vi "Navigation plus.vi"(11 "Array":dbl[](array[numeric])) -> (2 "length":i32, 3 "String":string)   [LabVIEW 2021]
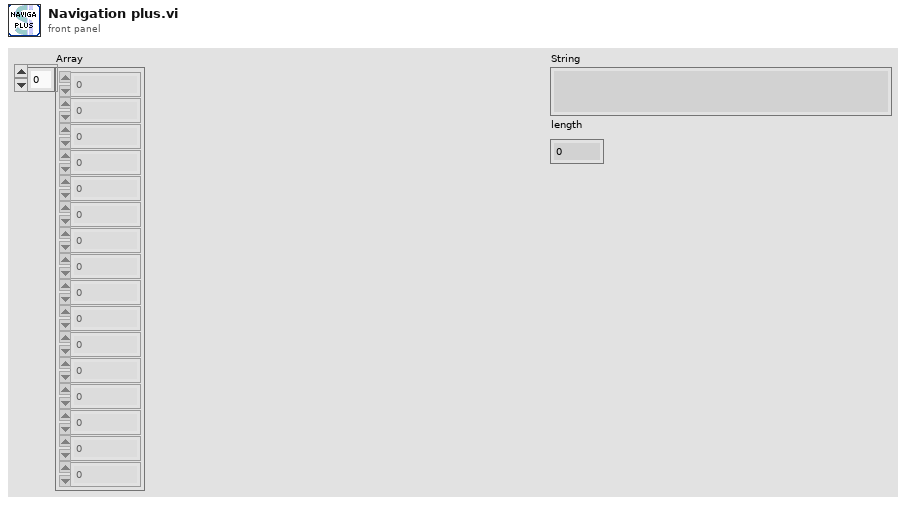
[diagram p1: front panel]
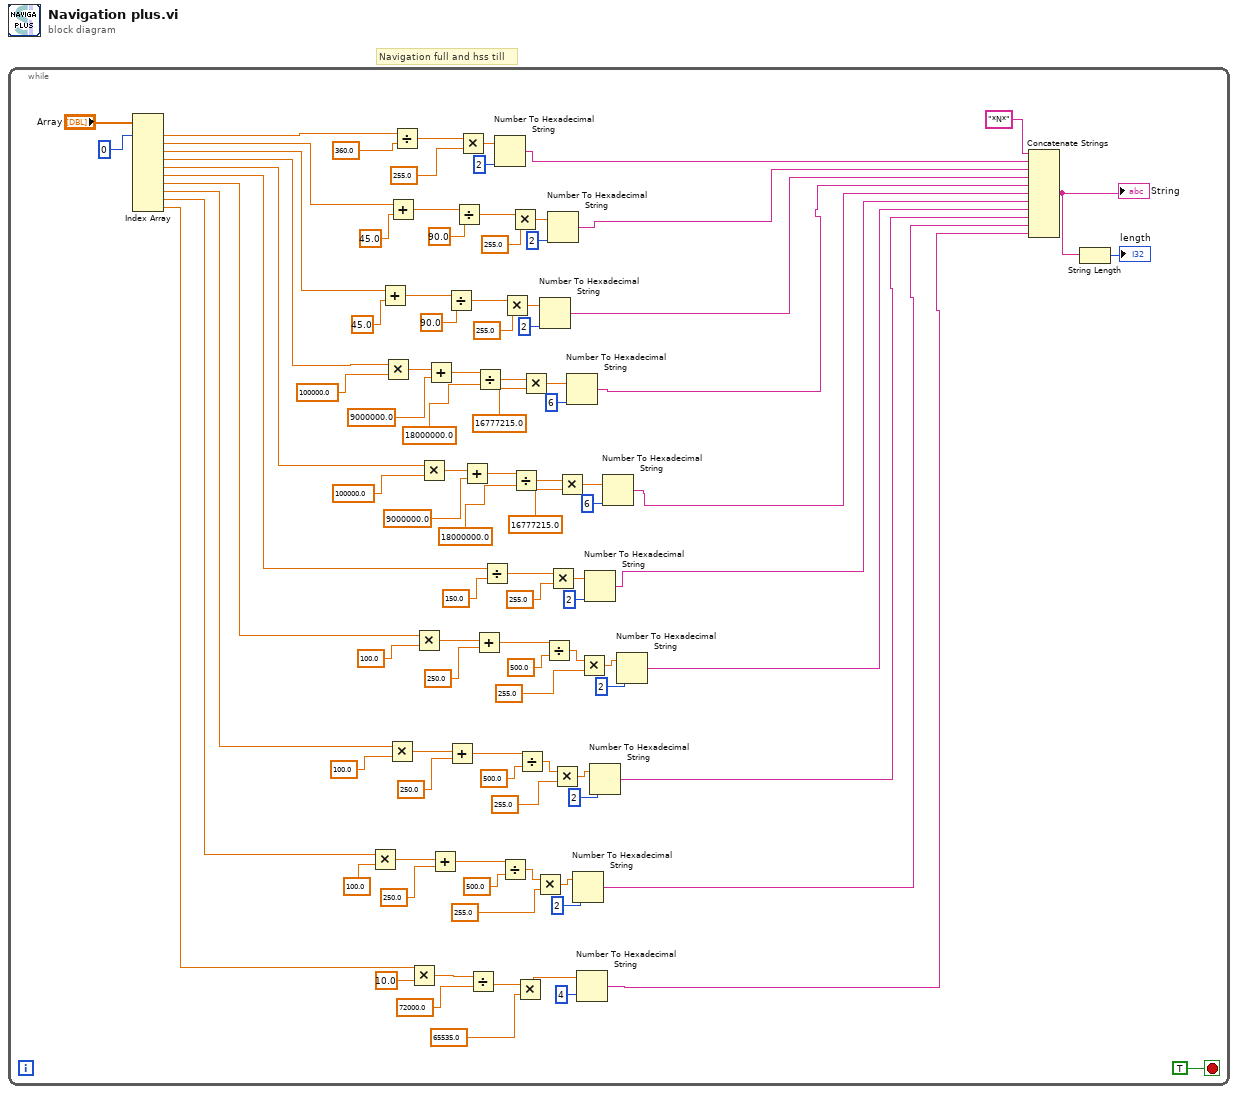
[diagram p0: block diagram]
diagram:
  # "Navigation full and hss till"
  n1 = while {
    stop <- TRUE stop-if-true
    n2 = Index Array(array="Array", index #1=0 ("index")) -> (element #1=w5:dbl, element #2=w24:dbl, element #3=w25:dbl, element #4=w34:dbl, element #5=w43:dbl, element #6=w48:dbl, element #7=w72:dbl, element #8=w73:dbl, element #9=w74:dbl, element #10=w80:dbl)  [unwired: 9 in]
    n3 = Multiply(x=w74, y=100.0) -> (x*y=w52:dbl)
    n4 = Add(x=w25, y=45.0) -> (x+y=w18:dbl)
    n5 = Multiply(x=w34, y=100000.0) -> (x*y=w26:dbl)
    n6 = Multiply(x=w73, y=100.0) -> (x*y=w67:dbl)
    n7 = Add(x=w24, y=45.0) -> (x+y=w12:dbl)
    n8 = Divide(x=w5, y=360.0) -> (x/y=w9:dbl)
    n9 = Multiply(x=w80, y=10.0) -> (x*y=w75:dbl)
    n10 = Multiply(x=w72, y=100.0) -> (x*y=w60:dbl)
    n11 = Multiply(x=w43, y=100000.0) -> (x*y=w35:dbl)
    n12 = Add(x=w26, y=9000000.0) -> (x+y=w29:dbl)
    n13 = Add(x=w52, y=250.0) -> (x+y=w49:dbl)
    n14 = Divide(x=w18, y=90.0) -> (x/y=w19:dbl)
    n15 = Add(x=w67, y=250.0) -> (x+y=w64:dbl)
    n16 = Divide(x=w12, y=90.0) -> (x/y=w13:dbl)
    n17 = Multiply(x=w9, y=255.0) -> (x*y=w10:dbl)
    n18 = Add(x=w35, y=9000000.0) -> (x+y=w38:dbl)
    n19 = Divide(x=w75, y=72000.0) -> (x/y=w77:dbl)
    n20 = Add(x=w60, y=250.0) -> (x+y=w57:dbl)
    n21 = Divide(x=w29, y=18000000.0) -> (x/y=w28:dbl)
    n22 = Divide(x=w48, y=150.0) -> (x/y=w45:dbl)
    n23 = Number To Hexadecimal String(1:i16 2 ("width (-)"), 2:w10) -> (0:w82:string)
    n24 = Divide(x=w49, y=500.0) -> (x/y=w50:dbl)
    n25 = Multiply(x=w19, y=255.0) -> (x*y=w20:dbl)
    n26 = Multiply(x=w13, y=255.0) -> (x*y=w14:dbl)
    n27 = Divide(x=w38, y=18000000.0) -> (x/y=w37:dbl)
    n28 = Multiply(x=w77, y=65535.0) -> (x*y=w76:dbl)
    n29 = Divide(x=w64, y=500.0) -> (x/y=w65:dbl)
    n30 = Multiply(x=w28, y=16777215.0) -> (x*y=w27:dbl)
    n31 = Multiply(x=w50, y=255.0) -> (x*y=w51:dbl)
    n32 = Number To Hexadecimal String(1:i16 2 ("width (-)"), 2:w20) -> (0:w95:string)
    n33 = Divide(x=w57, y=500.0) -> (x/y=w58:dbl)
    n34 = Number To Hexadecimal String(1:i16 2 ("width (-)"), 2:w14) -> (0:w94:string)
    n35 = Multiply(x=w45, y=255.0) -> (x*y=w44:dbl)
    n36 = Multiply(x=w65, y=255.0) -> (x*y=w66:dbl)
    n37 = Multiply(x=w37, y=16777215.0) -> (x*y=w36:dbl)
    n38 = Number To Hexadecimal String(1:i16 6 ("width (-)"), 2:w27) -> (0:w96:string)
    n39 = Number To Hexadecimal String(1:i16 2 ("width (-)"), 2:w51) -> (0:w101:string)
    n40 = Number To Hexadecimal String(1:i16 4 ("width (-)"), 2:w76) -> (0:w102:string)
    n41 = Multiply(x=w58, y=255.0) -> (x*y=w59:dbl)
    n42 = Number To Hexadecimal String(1:i16 2 ("width (-)"), 2:w44) -> (0:w98:string)
    n43 = Number To Hexadecimal String(1:i16 2 ("width (-)"), 2:w66) -> (0:w100:string)
    n44 = Number To Hexadecimal String(1:i16 6 ("width (-)"), 2:w36) -> (0:w97:string)
    n45 = Number To Hexadecimal String(1:i16 2 ("width (-)"), 2:w59) -> (0:w99:string)
    n46 = Concatenate Strings("*N*" ("string"), w82, w94, w95, w96, w97, w98, w99, w100, w101, w102) -> (w4:string)
    "String" <- w4
    n47 = String Length(string=w4) -> (length=→"length":i32)
  }
